vi "Append Image to Rich Text Box.vi"(8 "error in (no error)":errorcluster, 10 "Image File Path":path, 11 ".NET Refnum in":refnum<k24>) -> (0 "error out":errorcluster, 2 "Rtf Content":string)   [LabVIEW 2021, in "Rich Text Box.lvlib"]
uses:
  Rich Text Box.lvlib
  System.Windows.Forms
  System.Drawing
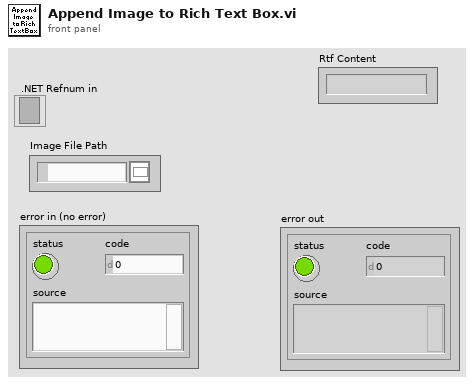
[diagram p1: front panel]
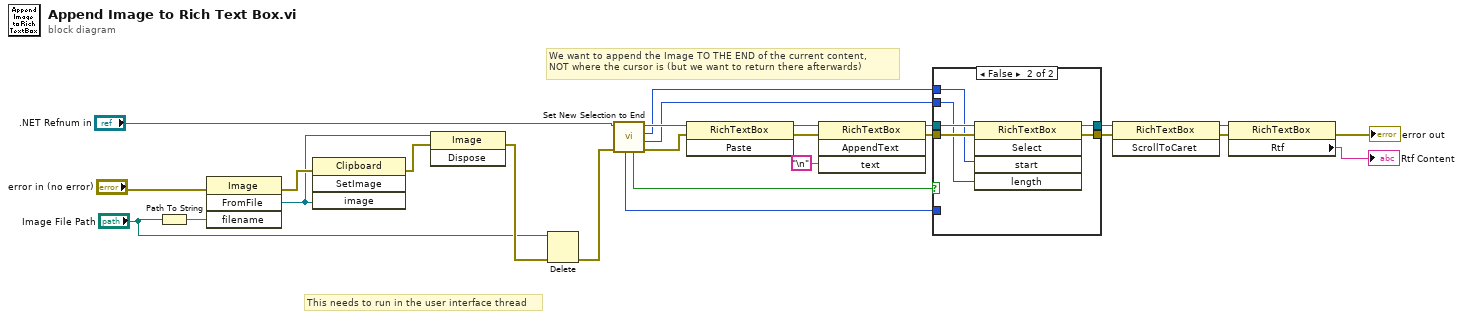
[diagram p0: block diagram]
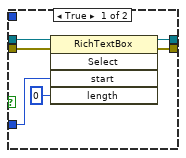
[diagram p2: hidden frame]
diagram:
  # "We want to append the Image TO THE END of the current content,\nNOT where the cursor is (but we want to return there afterwards)"
  # "This needs to run in the user interface thread"
  n1 = Path To String(path="Image File Path") -> (string=w22:string)
  n2 = invoke class="Image" method="FromFile"(error in="error in (no error)", "filename"=w22) -> (error out=w21:errorcluster, "FromFile"=w19:refnum<k24>)  [unwired: 2 in, 2 out]
  n3 = invoke class="Clipboard" method="SetImage"(error in=w21, "image"=w19) -> (error out=w18:errorcluster)  [unwired: 2 in, 3 out]
  n4 = invoke class="Image" method="Dispose"(reference=w19, error in=w18) -> (error out=w17:errorcluster)  [unwired: 1 in, 2 out]
  n5 = Delete(path (use dialog)="Image File Path", error in=w17) -> (error out=w14:errorcluster)  [unwired: 3 in, 2 out]
  n6 = call "Set New Selection to End.vi"("error in (no error)"=w14, ".NET Refnum in"=".NET Refnum in") -> ("error out"=w12:errorcluster, "Current SelectionLength"=w5:i32, "Current SelectionStart"=w4:i32, ".NET Refnum out"=w13:refnum<k24>, "Current Selection at End?"=w7:bool, "New SelectionStart: End of RTB"=w6:i32)  [unwired: 4 in]
  n7 = invoke class="RichTextBox" method="Paste"(reference=w13, error in=w12) -> (reference out=w26:refnum<k24>, error out=w25:errorcluster)  [unwired: 1 in, 1 out]
  n8 = invoke class="RichTextBox" method="AppendText"(reference=w26, error in=w25, "text"="\n") -> (reference out=w11:refnum<k24>, error out=w10:errorcluster)  [unwired: 1 in, 2 out]
  n9 = case shown="False" w7 {
    tunnel: w11 -> [w32 w38]
    tunnel: w10 -> [w31 w37]
    tunnel: [w30 w36] -> w9
    tunnel: [w29 w35] -> w8
    tunnel: w6 -> [w27 _]
    tunnel: w5 -> [_ w34]
    tunnel: w4 -> [_ w33]
    frame True {
      n10 = invoke class="RichTextBox" method="Select"(reference=w32, error in=w31, "start"=w27, "length"=0) -> (reference out=w30:refnum<k24>, error out=w29:errorcluster)  [unwired: 1 in, 3 out]
    }
    frame False {
      n11 = invoke class="RichTextBox" method="Select"(reference=w38, error in=w37, "start"=w33, "length"=w34) -> (reference out=w36:refnum<k24>, error out=w35:errorcluster)  [unwired: 1 in, 3 out]
    }
  }
  n12 = invoke class="RichTextBox" method="ScrollToCaret"(reference=w9, error in=w8) -> (reference out=w2:refnum<k24>, error out=w20:errorcluster)  [unwired: 1 in, 1 out]
  n13 = property class="RichTextBox"(reference=w2, error in=w20) -> (error out=→"error out":errorcluster, "Rtf"=→"Rtf Content":string)  [unwired: 1 out]
